vi "LidarLiteV3_Counter_Sample.vi"() -> ()   [LabVIEW 2020]
uses:
  <vilib>/Rock Robotics/SystemInterfaces/DIO/FPGA_DIOChannel.ctl
  <vilib>/Rock Robotics/WPI/Counter/WPI_CounterDigitalInputToDigitalSource.vi
  <vilib>/Rock Robotics/WPI/Counter/WPI_CounterOpen Semi Period Mode.vi
  <vilib>/ptbypt/NI_PtbyPt.lvlib
panel:
  in  "Hardware Number \nSamples to Average":u8=25
  in  "Average FIlter\nSamples":i32=20
  in  "Calibration\nOffset":dbl format="%#_13g"
  in  "Calibration \nGain":dbl=1.0 format="%#_13g"
  out "Lidar Distance Chart":cluster{dbl, "mean":dbl}(graph)
  out "Distance\nAverage FIlter\nFeet":dbl format="%19.3f"
  out "Period\nMicroSeconds":dbl format="%22.1f"
  out "Distance\nFeet":dbl format="%19.3f"
  in  "High Pulse (T)":bool=TRUE
  in  "PWM (Counter) Input":T1=enum."DIO 3"
  # "Read Lidar Lite V3 Using PWM  (Counter)"
  # "Set these values before\nexecuting program"
  # "These values can be\nchanged while the \nprogram is running"
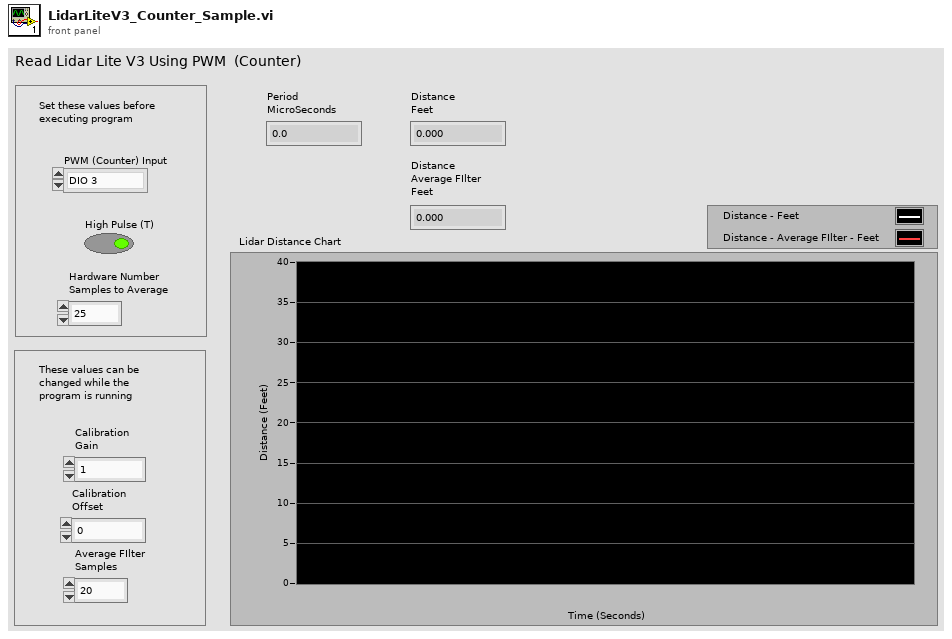
[diagram p1: front panel]
types:
  T1 = typedef "FPGA_DIOChannel.ctl" = enum8{"DIO 0", "DIO 1", "DIO 2", "DIO 3", "DIO 4", "DIO 5", "DIO 6", "DIO 7", "DIO 8", "DIO 9", "DIO MXP 0", "DIO MXP 1", "DIO MXP 2", "DIO MXP 3", "DIO MXP 4", "DIO MXP 5", "DIO MXP 6", "DIO MXP 7", "DIO MXP 8", "DIO MXP 9", "DIO MXP 10", "DIO MXP 11", "DIO MXP 12", "DIO MXP 13", "DIO MXP 14", "DIO MXP 15", "SPI Port CS1", "SPI Port CS2", "SPI Port CS3", "SPI Port MISO", "SPI Port MOSI", "Invalid"}
  T2 = typedef "WPI_DigitalInputDevRef.ctl" = cluster{"DevStatus":errorcluster, "DIO Channel":T1}
  T3 = typedef "FPGA_CounterEncoderSourceConvertionLVSourceType.ctl" = cluster{"DevStatus":errorcluster, "AnalogTriggerMode?":bool, "DigitalMode":cluster{"DIO Channel":T4}, "AnalogTriggerMode":cluster{"AnalogTriggerIndex":T5, "OutputType":T6}}
  T4 = typedef "FPGA_DIODigitalSourceChannel.ctl" = enum8{"DIO 0", "DIO 1", "DIO 2", "DIO 3", "DIO 4", "DIO 5", "DIO 6", "DIO 7", "DIO 8", "DIO 9", "DIO MXP 0", "DIO MXP 1", "DIO MXP 2", "DIO MXP 3", "DIO MXP 4", "DIO MXP 5", "DIO MXP 6", "DIO MXP 7", "DIO MXP 8", "DIO MXP 9", "DIO MXP 10", "DIO MXP 11", "DIO MXP 12", "DIO MXP 13", "DIO MXP 14", "DIO MXP 15", "SPI Port CS1", "SPI Port CS2", "SPI Port CS3", "SPI Port MISO", "SPI Port MOSI", "Disabled"}
  T5 = typedef "FPGA_AnalogTriggerIndex.ctl" = enum8{"Trig 0", "Trig 1", "Trig 2", "Trig 3", "Trig 4", "Trig 5", "Trig 6", "Trig 7", "Invalid"}
  T6 = typedef "FPGA_AnalogTriggerOutType.ctl" = enum16{"InWindow", "TriggerState", "Rising", "Falling"}
  T7 = typedef "WPI_CounterDevRef.ctl" = cluster{"DevStatus":errorcluster, "CntIndex":T8}
  T8 = typedef "FPGA_CounterCtrSystemIndex.ctl" = enum8{"Ctr 0", "Ctr 1", "Ctr 2", "Ctr 3", "Ctr 4", "Ctr 5", "Ctr 6", "Ctr 7", "Invalid"}
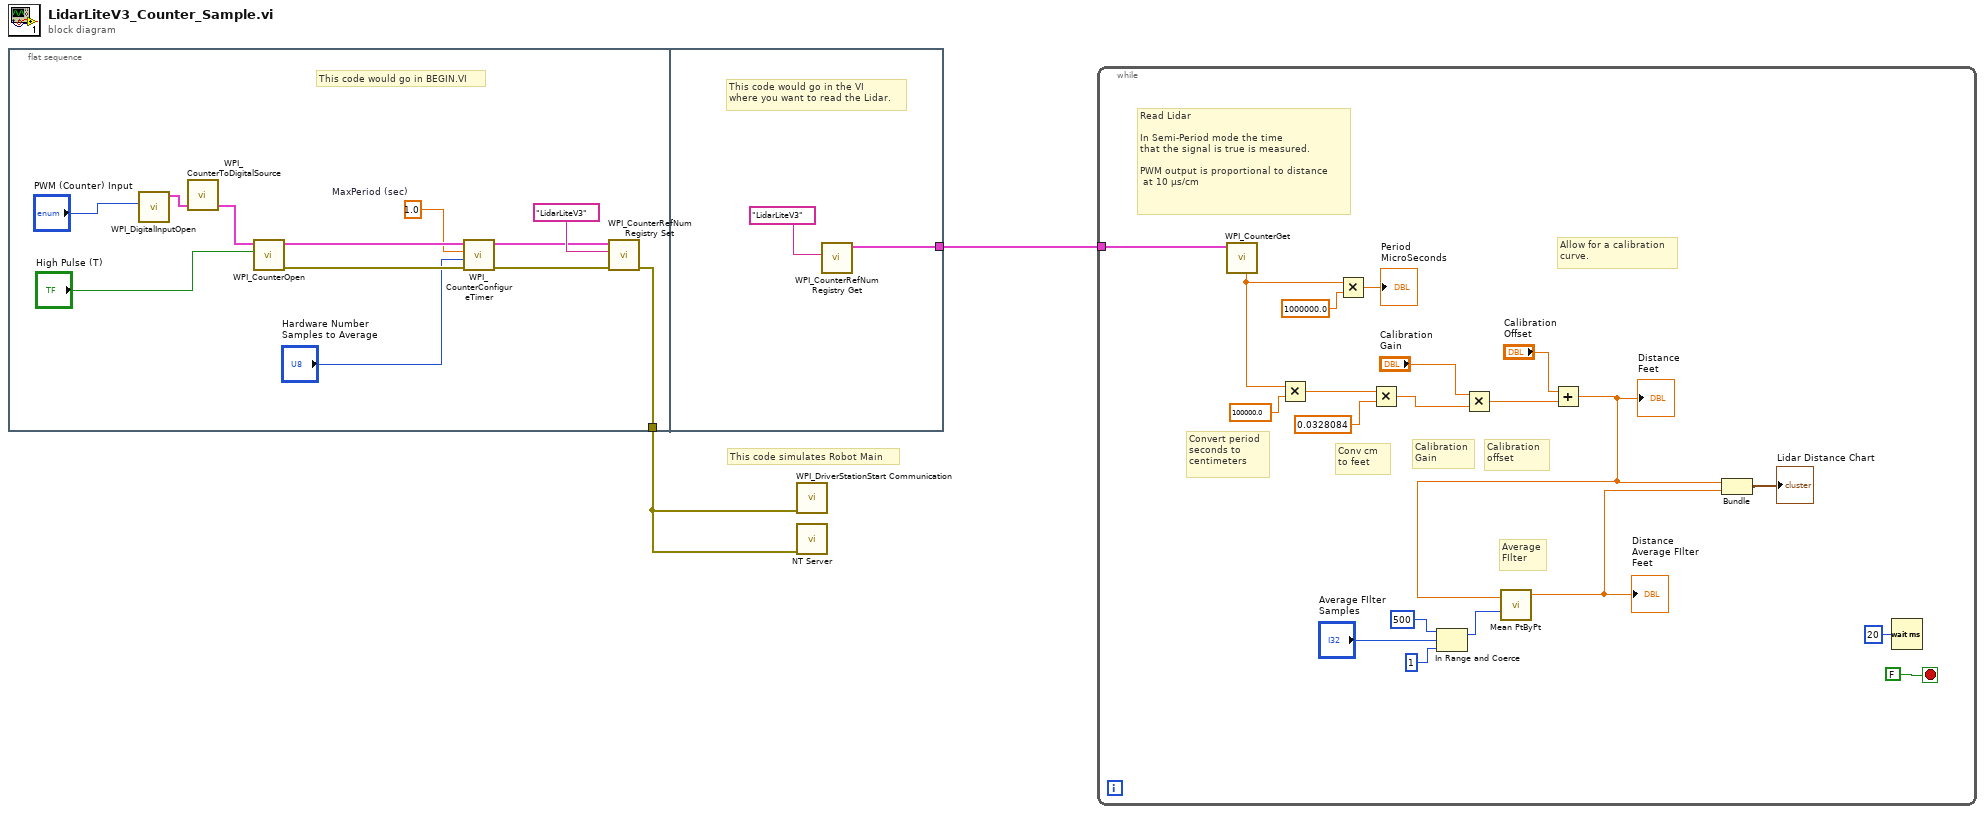
[diagram p0: block diagram]
diagram:
  # "This code simulates Robot Main"
  n1 = flat-sequence {
    tunnel: [w3] -> w1
    tunnel: [w15] -> w2
    frame #0 {
      w4 = 1.0  # MaxPeriod (sec)
      # "This code would go in BEGIN.VI"
      n2 = call <vilib>:"WPI_DigitalInputOpen.vi"("DIO Channel"="PWM (Counter) Input") -> ("DigitalInputDevRef"=w12:T2)  [unwired: 1 in, 9 out]
      n3 = call-poly <vilib>:"WPI_CounterToDigitalSource.vi"("DigitalInputDevRef"=w12) -> ("Digital Source"=w14:T3)  [unwired: 6 out]
      n4 = call-poly <vilib>:"WPI_CounterOpen.vi"("High Pulse (T)"="High Pulse (T)", "Source"=w14) -> ("error out"=w8:errorcluster, "CounterDevRef"=w9:T7)  [unwired: 3 in, 5 out]
      n5 = call <vilib>:"WPI_CounterConfigureTimer.vi"("error in (no error)"=w8, "Number Samples to Average"="Hardware Number \nSamples to Average", "MaxPeriod (sec)"=w4, "CounterDevRef in"=w9) -> ("error out"=w7:errorcluster, "CounterDevRef out"=w6:T7)  [unwired: 6 in]
      n6 = call <vilib>:"WPI_CounterRefNum Registry Set.vi"("error in (no error)"=w7, "refnum name"="LidarLiteV3", "CounterDevRef"=w6) -> ("error out"=w3:errorcluster)  [unwired: 7 in, 1 out]
    }
    frame #1 {
      # "This code would go in the VI\nwhere you want to read the Lidar."
      n7 = call <vilib>:"WPI_CounterRefNum Registry Get.vi"("refnum name"="LidarLiteV3") -> ("CounterDevRef"=w15:T7)  [unwired: 9 in, 1 out]
    }
  }
  n8 = call <vilib>:"WPI_DriverStationStart Communication.vi"("error in (no error)"=w1) -> ()  [unwired: 11 in]
  n9 = call <vilib>:"NT Server.vi"("error in (no error)"=w1) -> ()  [unwired: 11 in]
  n10 = while {
    tunnel: w2 -> [w31]
    stop <- FALSE stop-if-true
    # "Average\nFIlter"
    # "Allow for a calibration\ncurve."
    # "Convert period\nseconds to\ncentimeters"
    # "Read Lidar\n\nIn Semi-Period mode the time\nthat the signal is true is measured.\n\nPWM output is proportional to distance\n at 10 µs/cm"
    # "Calibration\nGain"
    # "Conv cm \nto feet"
    # "Calibration \noffset"
    n11 = call <vilib>:"WPI_CounterGet.vi"("CounterDevRef in"=w31) -> ("Period (sec)"=w29:dbl)  [unwired: 5 in, 5 out]
    n12 = Multiply(x=w29, y=100000.0) -> (x*y=w34:dbl)
    n13 = Multiply(x=w29, y=1000000.0) -> (x*y=→"Period\nMicroSeconds":dbl)
    n14 = Multiply(x=w34, y=0.0328084) -> (x*y=w24:dbl)
    n15 = In Range and Coerce(upper limit=500, x="Average FIlter\nSamples", lower limit=1) -> (coerced(x)=w17:i32)  [unwired: 1 out]
    n16 = Multiply(x="Calibration \nGain", y=w24) -> (x*y=w22:dbl)
    n17 = Add(x="Calibration\nOffset", y=w22) -> (x+y=w26:dbl)
    "Distance\nFeet" <- w26
    n18 = call <vilib>:"Mean PtByPt.vi"("x"=w26, "sample length"=w17) -> ("mean"=w25:dbl)  [unwired: 2 in, 1 out]
    "Distance\nAverage FIlter\nFeet" <- w25
    n19 = Bundle(w26, "mean"=w25) -> (→"Lidar Distance Chart":cluster{dbl, "mean":dbl})  [unwired: 1 in]
    n20 = Wait (ms)(milliseconds to wait=u32 20) -> ()  [unwired: 1 out]
  }
